vi "practica 1.vi"() -> ()   [LabVIEW 2014]
panel:
  in  "Stop Button":bool
  in  "Cluster":T1 {"AMPLITUD" scale=0.0..10.0; "FRECUENCIA" scale=0.0..100.0}
  out "Waveform Chart":dynamicdata(graph)
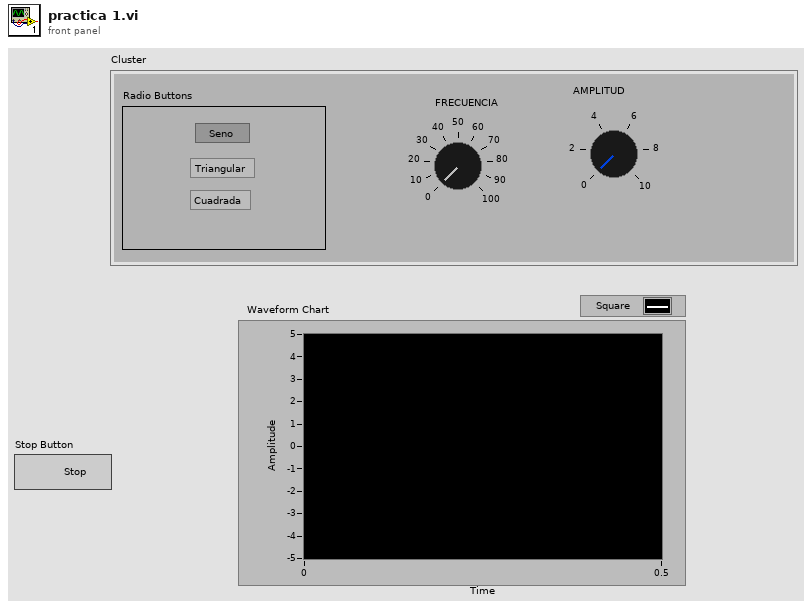
[diagram p1: front panel]
types:
  T1 = cluster{"FRECUENCIA":dbl, "AMPLITUD":dbl, "Radio Buttons":enum32{"Seno", "Triangular", "Cuadrada"}}
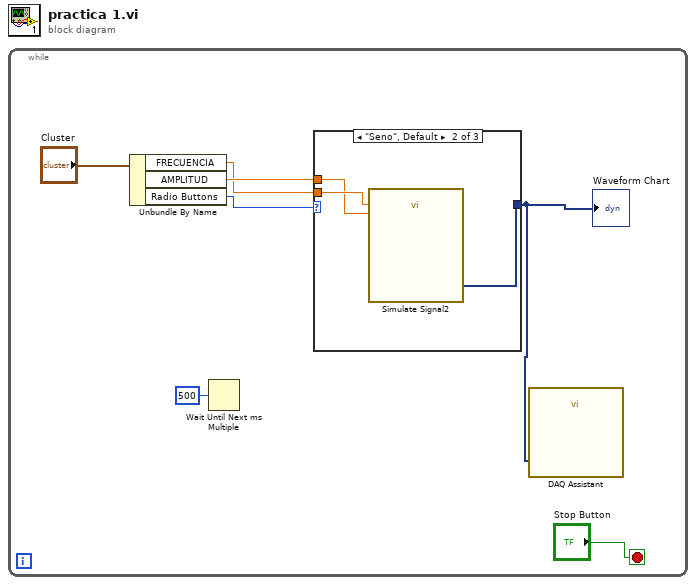
[diagram p0: block diagram]
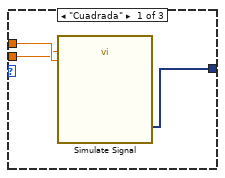
[diagram p2: hidden frame]
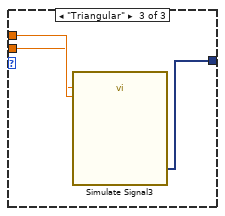
[diagram p3: hidden frame]
diagram:
  n1 = while {
    stop <- "Stop Button" stop-if-true
    n2 = Unbundle By Name("Cluster") -> ("FRECUENCIA"=w3:dbl, "AMPLITUD"=w4:dbl, "Radio Buttons"=w5:enum32{"Seno", "Triangular", "Cuadrada"})
    n3 = Wait Until Next ms Multiple(millisecond multiple=u32 500) -> ()  [unwired: 1 out]
    n4 = case shown="\"Seno\", Default" w5 {
      tunnel: w4 -> [w10 w12 w16]
      tunnel: w3 -> [w9 w13 w15]
      tunnel: [w8 w11 w14] -> w1
      frame "Cuadrada" {
        n5 = call "Simulate Signal"("Frequency"=w9, "Amplitude"=w10) -> ("Square"=w8:dynamicdata)  [unwired: 12 in, 1 out]
      }
      frame "Seno", Default {
        n6 = call "Simulate Signal2"("Frequency"=w13, "Amplitude"=w12) -> ("Sine"=w11:dynamicdata)  [unwired: 12 in, 1 out]
      }
      frame "Triangular" {
        n7 = call "Simulate Signal3"("Frequency"=w15, "Amplitude"=w16) -> ("Triangle"=w14:dynamicdata)  [unwired: 12 in, 1 out]
      }
    }
    "Waveform Chart" <- w1
    n8 = call "DAQ Assistant"("data"=w1) -> ()  [unwired: 16 in, 3 out]
  }
